vi "Cal IC (Numeric).vi"(8 "error in (no error)":errorcluster, 10 "IC in":variant, 11 "Domain_Evolut_2D_Rect in":refnum<class "NI_Domain_Evolut_2D_Rect.lvclass">) -> (0 "error out":errorcluster, 2 "IC out":variant, 3 "Domain_Evolut_2D_Rect out":refnum<class "NI_Domain_Evolut_2D_Rect.lvclass">)   [LabVIEW 2020, in "NI_PDE.lvlib" / "NI_Domain_Evolut_2D_Rect.lvclass"]
uses:
  <vilib>/gmath/pde.llb/DomainClass/Domain_Evolut_2D_Rect/NI_Domain_Evolut_2D_Rect.lvclass
  <vilib>/gmath/pde.llb/ICClass/IC_2D_Numeric/IC Data.ctl
  <vilib>/gmath/pde.llb/Common/PDE_IC Type.ctl
  <vilib>/gmath/pde.llb/DomainClass/Domain_Evolut_2D_Rect/NI_Domain_Evolut_2D_Rect.lvclass/NI_Domain_Evolut_2D_Rect.ctl
  <vilib>/gmath/NI_PDE.lvlib
  <vilib>/gmath/pde.llb/ICClass/IC_2D_Numeric/NI_IC_2D_Numeric.lvclass
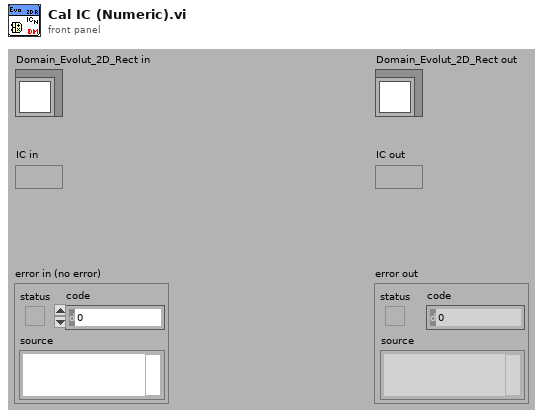
[diagram p1: front panel]
types:
  T1 = typedef "NI_PDE.lvlib/NI_IC_2D_Numeric.lvclass/IC Data.ctl" = cluster{"type":T2, "H":dbl[][]}
  T2 = typedef "NI_PDE.lvlib/PDE_IC Type.ctl" = i32
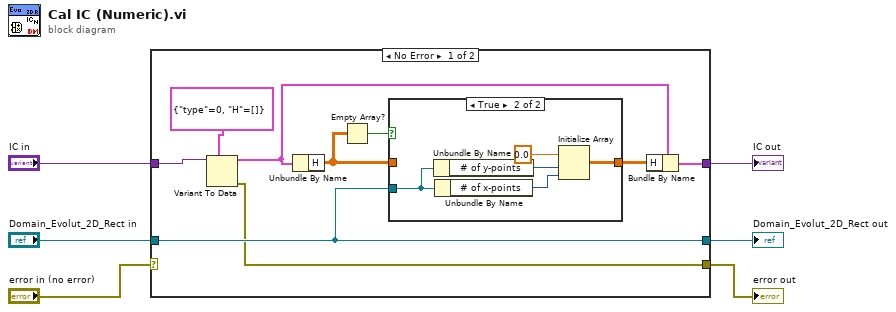
[diagram p0: block diagram]
diagram:
  n1 = case shown="No Error" "error in (no error)" {
    selector: "error in (no error)" -> [_ w24]
    tunnel: "Domain_Evolut_2D_Rect in" -> [w8 w23]
    tunnel: [w8 w23] -> w6
    tunnel: [w7 w24] -> w5
    tunnel: [w13 w22] -> w2
    tunnel: "IC in" -> [w15 w22]
    frame No Error {
      n2 = Variant To Data(type=T1 {"type"=0, "H"=[]} ("IC data"), Variant=w15) -> (data=w14:T1, error out=w7:errorcluster)  [unwired: 1 in]
      n3 = Unbundle By Name(w14) -> ("H"=w10:dbl[][])
      n4 = Empty Array?(array=w10) -> (empty?=w11:bool)
      n5 = case shown="True" w11 {
        tunnel: w8 -> [_ w17]
        tunnel: w10 -> [w16 _]
        tunnel: [w16 w21] -> w9
        frame False {
        }
        frame True {
          n6 = Unbundle By Name(w17) -> ("# of y-points"=w19:i32)
          n7 = Unbundle By Name(w17) -> ("# of x-points"=w18:i32)
          n8 = Initialize Array(0.0 ("element"), w19, w18) -> (w21:dbl[][])
        }
      }
      n9 = Bundle By Name(cluster=w14, "H"=w9) -> (w13:T1)
    }
    frame Error {
    }
  }
  "Domain_Evolut_2D_Rect out" <- w6
  "error out" <- w5
  "IC out" <- w2
